vi "AnalyzeLowUpdateData.vi"(8 "error in (no error)":errorcluster, 9 "data in":T12, 11 "Analysis Configuration In":T1 {"Groups"."Calculation Cache"."speed initial conditions"."zoom FFT settings"."FFT settings"."window" items=["Rectangle"=0, "Hanning"=1, "Hamming"=2, "Blackman-Harris"=3, "Exact Blackman"=4, "Blackman"=5, "Flat Top"=6, "4 Term B-Harris "=7, "7 Term B-Harris"=8, "Low Sidelobe"=9, "Blackman Nuttall"=11, "Triangle"=30, "Bartlett-Hanning"=31, "Bohman"=32, "Parzen"=33, "Welch"=34, "Kaiser"=60, "Dolph-Chebyshev"=61, "Gaussian"=62]; "Groups"."Calculation Cache"."spectrum initial conditions"."zoom FFT settings"."FFT settings"."window" items=["Rectangle"=0, "Hanning"=1, "Hamming"=2, "Blackman-Harris"=3, "Exact Blackman"=4, "Blackman"=5, "Flat Top"=6, "4 Term B-Harris "=7, "7 Term B-Harris"=8, "Low Sidelobe"=9, "Blackman Nuttall"=11, "Triangle"=30, "Bartlett-Hanning"=31, "Bohman"=32, "Parzen"=33, "Welch"=34, "Kaiser"=60, "Dolph-Chebyshev"=61, "Gaussian"=62]}) -> (0 "error out":errorcluster, 1 "data out":T12, 3 "Analysis Configuration Out":T1 {"Groups"."Calculation Cache"."speed initial conditions"."zoom FFT settings"."FFT settings"."window" items=["Rectangle"=0, "Hanning"=1, "Hamming"=2, "Blackman-Harris"=3, "Exact Blackman"=4, "Blackman"=5, "Flat Top"=6, "4 Term B-Harris "=7, "7 Term B-Harris"=8, "Low Sidelobe"=9, "Blackman Nuttall"=11, "Triangle"=30, "Bartlett-Hanning"=31, "Bohman"=32, "Parzen"=33, "Welch"=34, "Kaiser"=60, "Dolph-Chebyshev"=61, "Gaussian"=62]; "Groups"."Calculation Cache"."spectrum initial conditions"."zoom FFT settings"."FFT settings"."window" items=["Rectangle"=0, "Hanning"=1, "Hamming"=2, "Blackman-Harris"=3, "Exact Blackman"=4, "Blackman"=5, "Flat Top"=6, "4 Term B-Harris "=7, "7 Term B-Harris"=8, "Low Sidelobe"=9, "Blackman Nuttall"=11, "Triangle"=30, "Bartlett-Hanning"=31, "Bohman"=32, "Parzen"=33, "Welch"=34, "Kaiser"=60, "Dolph-Chebyshev"=61, "Gaussian"=62]})   [LabVIEW 2017, in "McsaAnalysisLowUpdate.lvlib"]
uses:
  <vilib>/addons/InsightCM/Devices/Shared/Mcsa/McsaAnalysisLowUpdate/McsaAnalysisLowUpdate.lvlib
  <vilib>/addons/InsightCM/Devices/Shared/Common/DataFlow/controls/Data.ctl
  <vilib>/addons/InsightCM/Utilities/DataAccessors/controls/wfmSGL_DVR.ctl
  <vilib>/addons/PointValueMap/controls/PointMap.ctl
  <vilib>/addons/InsightCM/Devices/Shared/Common/DataFlow/controls/Type.ctl
  <vilib>/addons/InsightCM/Devices/Shared/Mcsa/McsaAnalysisLowUpdate/controls/Config.ctl
  <vilib>/addons/InsightCM/Devices/Shared/Mcsa/McsaAnalysisLowUpdate/controls/Group.ctl
  <vilib>/addons/InsightCM/Utilities/Analysis/MCSA/controls/McsaLowUpdateChannel.ctl
  <vilib>/addons/InsightCM/Utilities/Analysis/Shared/controls/Feature.ctl
  <vilib>/addons/InsightCM/Utilities/Analysis/Shared/controls/AmplitudeScale.ctl
  <vilib>/addons/InsightCM/Utilities/Analysis/MCSA/controls/McsaMotor.ctl
  <vilib>/addons/InsightCM/Utilities/Analysis/MCSA/controls/McsaCalculationCache.ctl
  <vilib>/addons/Electrical Power/Motor Monitoring/subVIs/ep_Initial Conditions for MCSA Spectra.ctl
  <vilib>/addons/Electrical Power/Motor Monitoring/subVIs/ep_Demodulation Algorithm.ctl
  <vilib>/addons/Electrical Power/Motor Monitoring/subVIs/ep_Zoom FFT Settings.ctl
  <vilib>/addons/Electrical Power/Motor Monitoring/subVIs/ep_Initial Conditions for Speed Estimation.ctl
  <vilib>/addons/InsightCM/Devices/Shared/Mcsa/McsaResourceScheduler/McsaResourceScheduler.lvlib
  <vilib>/addons/PointValueMap/PointValueMap.lvlib
  <vilib>/addons/InsightCM/Devices/Shared/Common/DataFlow/DataFlow.lvlib
  <vilib>/addons/InsightCM/Utilities/Analysis/Shared/AnalysisHelper.lvlib
  <vilib>/addons/InsightCM/Utilities/Analysis/MCSA/McsaAnalysisFunctions.lvlib
  <vilib>/addons/Electrical Power/Motor Monitoring/NI_EP_Motor Monitoring.lvlib
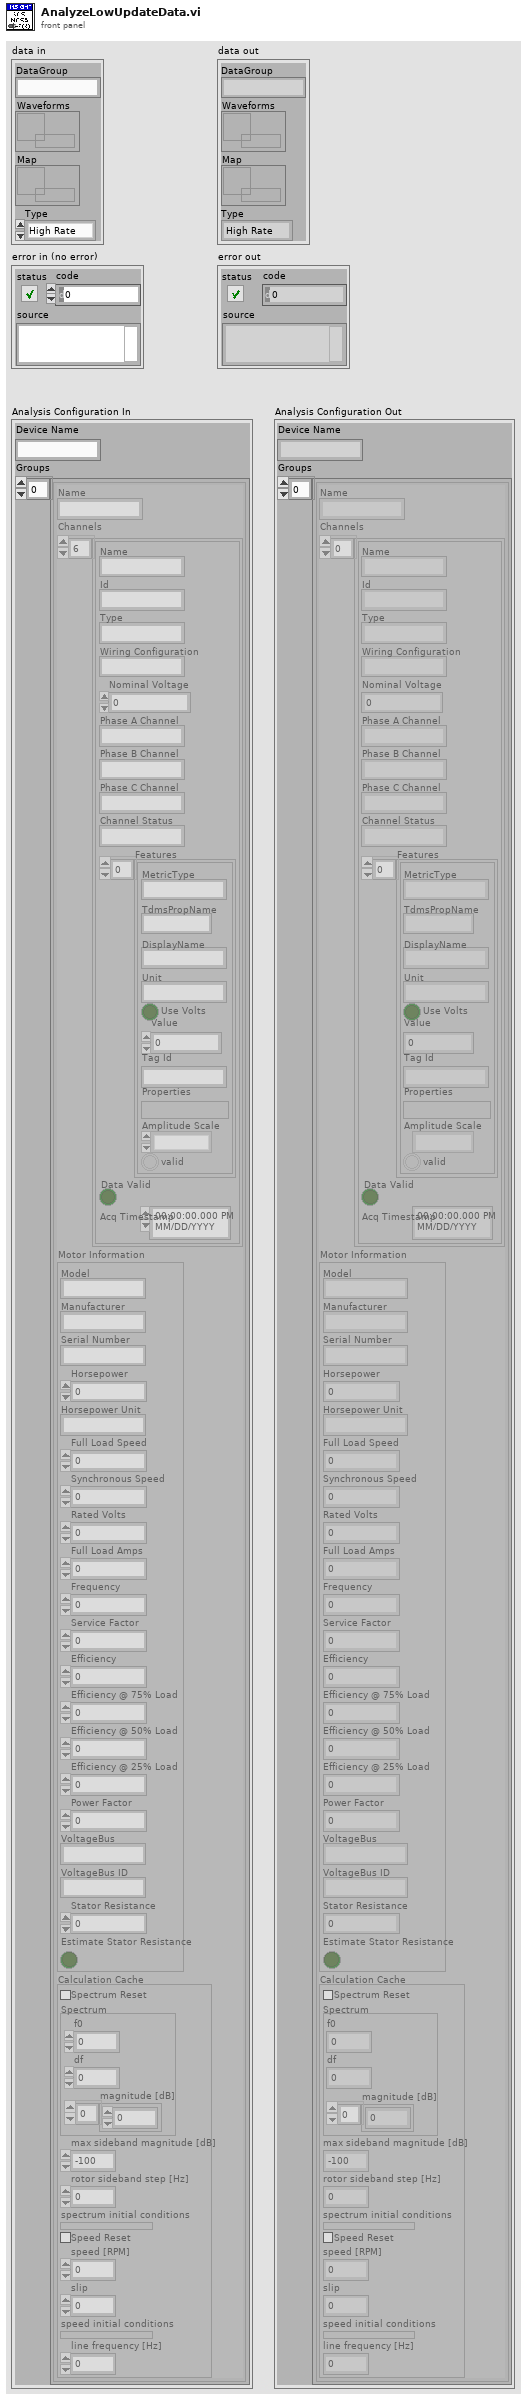
[diagram p1: front panel]
types:
  T1 = typedef "McsaAnalysisLowUpdate.lvlib/Config.ctl" = cluster{"Device Name":string, "Groups":T2[]}
  T2 = typedef "McsaAnalysisLowUpdate.lvlib/Group.ctl" = cluster{"Name":string, "Channels":T3[], "Motor Information":T6, "Calculation Cache":T7}
  T3 = typedef "McsaAnalysisFunctions.lvlib/McsaLowUpdateChannel.ctl" = cluster{"Name":string, "Id":string, "Type":string, "Wiring Configuration":string, "Nominal Voltage":dbl, "Phase A Channel":string, "Phase B Channel":string, "Phase C Channel":string, "Channel Status":string, "Features":T4[], "Data Valid":bool, "Acq Timestamp":timestamp}
  T4 = typedef "AnalysisHelper.lvlib/Feature.ctl" = cluster{"MetricType":string, "TdmsPropName":string, "DisplayName":string, "Unit":string, "Use Volts":bool, "Value":dbl, "Tag Id":string, "Properties":variant, "Amplitude Scale":T5, "valid":bool}
  T5 = typedef "AnalysisHelper.lvlib/AmplitudeScale.ctl" = enum16{"rms", "peak", "pk-pk"}
  T6 = typedef "McsaAnalysisFunctions.lvlib/McsaMotor.ctl" = cluster{"Model":string, "Manufacturer":string, "Serial Number":string, "Horsepower":dbl, "Horsepower Unit":string, "Full Load Speed":dbl, "Synchronous Speed":dbl, "Rated Volts":dbl, "Full Load Amps":dbl, "Frequency":dbl, "Service Factor":dbl, "Efficiency":dbl, "Efficiency @ 75% Load":dbl, "Efficiency @ 50% Load":dbl, "Efficiency @ 25% Load":dbl, "Power Factor":dbl, "VoltageBus":string, "VoltageBus ID":string, "Stator Resistance":dbl, "Estimate Stator Resistance":bool}
  T7 = typedef "McsaAnalysisFunctions.lvlib/McsaCalculationCache.ctl" = cluster{"Spectrum Reset":bool, "Spectrum":cluster{"f0":dbl, "df":dbl, "magnitude [dB]":dbl[]}, "max sideband magnitude [dB]":dbl, "rotor sideband step [Hz]":dbl, "spectrum initial conditions":T8, "Speed Reset":bool, "speed [RPM]":dbl, "slip":dbl, "speed initial conditions":T11, "line frequency [Hz]":dbl}
  T8 = typedef "NI_EP_Motor Monitoring.lvlib/ep_Initial Conditions for MCSA Spectra.ctl" = cluster{"hilbert state":cluster{"delay conditions":dbl[], "filter conditions":dbl[]}, "zoom FFT state":cluster{"phase state":dbl, "zoom FFT state":cluster{"zoom settings state":cluster{"zoom":i32, "stop band attenuation":enum16{"84 dB", "96 dB", "120 dB"}, "alias protect in final transition":bool, "oversampling ratio":dbl}, "SML Decimation Filter (complex input) state":cluster{"decimation settings state":cluster{"M":i32, "stop band attenuation":enum16{"84 dB", "96 dB", "120 dB"}, "alias protect in transition band":bool, "oversampling ratio":dbl}, "counter for garbage samples state":i32, "sml_Parameter Setting for Zoom Factor state":cluster{"filter length * interpolation state":i32, "interpolation state":i32, "comb filter order state":i32, "CFIR par state":cluster{"h":dbl[], "M":i32, "N":i32}, "LFIR par state":cluster{"h":dbl[], "M":i32, "N":i32}, "CIC Stages state":i32}, "aal_CIC (complex input) state":cluster{"aal_cascaded moving average (complex input) state":cluster{"states":cdb[], "circular buffers state":cdb[][], "circular buffer counter state":i32}, "aal_moving average with decimation by order (complex input) state":cluster{"residue result state":cdb, "processed data counter state":i32}}, "sml_Cascaded Decimation Filter (complex input) CFIR state":cluster{"unprocessed data state":cdb[], "final conditions state":cdb[][], "sml_M-1 Decimator with IC (complex input) state":cluster{"coefficients in reverse order state":dbl[], "max index for coefficients state":i32}}, "sml_Cascaded Decimation Filter (complex input) LFIR state":cluster{"unprocessed data state":cdb[], "final conditions state":cdb[][], "sml_M-1 Decimator with IC (complex input) state":cluster{"coefficients in reverse order state":dbl[], "max index for coefficients state":i32}}}, "ma_SML Data Packing (complex input) state":cluster{"array getting packed state":cdb[], "last array processed state":cdb[], "index state":i32, "packing parameters state":cluster{i32, "size":i32}}}, "FFT{X} [Vrms]":cdb[]}, "IIR filter state":cluster{"filter state":dbl[]}, "demodulation settings":cluster{"enable? (F)":bool, "algorithm":T9}, "highpass IIR Filter":cluster{"filter structure":enum32{"IIR 2nd Order", "IIR 4th Order"}, "Reverse Coefficients":dbl[], "Forward Coefficients":dbl[]}, "Hilbert FIR filter":cluster{"coefficients":dbl[], "delay":i32}, "zoom FFT settings":T10}
  T9 = typedef "NI_EP_Motor Monitoring.lvlib/ep_Demodulation Algorithm.ctl" = enum16{"1-phase signal", "3-phase signals"}
  T10 = typedef "NI_EP_Motor Monitoring.lvlib/ep_Zoom FFT Settings.ctl" = cluster{"FFT settings":cluster{"window":u16, "Window Size":i32, "FFT Size":i32, "%overlap":dbl}, "zoom settings":cluster{"zoom":i32, "stop band attenuation":enum16{"84 dB", "96 dB", "120 dB"}, "alias protect in final transition":bool, "oversampling ratio":dbl}, "other settings":cluster{"fmod":dbl, "f0":dbl, "df":dbl, "oidx":i32, "olen":i32}, "iterations":i32, "max block size":i32, "fs":dbl}
  T11 = typedef "NI_EP_Motor Monitoring.lvlib/ep_Initial Conditions for Speed Estimation.ctl" = cluster{"SVAF state":cluster{"space vector amplitude":dbl, "hilbert state":cluster{"delay conditions":dbl[], "filter conditions":dbl[]}}, "zoom FFT state":cluster{"phase state":dbl, "zoom FFT state":cluster{"zoom settings state":cluster{"zoom":i32, "stop band attenuation":enum16{"84 dB", "96 dB", "120 dB"}, "alias protect in final transition":bool, "oversampling ratio":dbl}, "SML Decimation Filter (complex input) state":cluster{"decimation settings state":cluster{"M":i32, "stop band attenuation":enum16{"84 dB", "96 dB", "120 dB"}, "alias protect in transition band":bool, "oversampling ratio":dbl}, "counter for garbage samples state":i32, "sml_Parameter Setting for Zoom Factor state":cluster{"filter length * interpolation state":i32, "interpolation state":i32, "comb filter order state":i32, "CFIR par state":cluster{"h":dbl[], "M":i32, "N":i32}, "LFIR par state":cluster{"h":dbl[], "M":i32, "N":i32}, "CIC Stages state":i32}, "aal_CIC (complex input) state":cluster{"aal_cascaded moving average (complex input) state":cluster{"states":cdb[], "circular buffers state":cdb[][], "circular buffer counter state":i32}, "aal_moving average with decimation by order (complex input) state":cluster{"residue result state":cdb, "processed data counter state":i32}}, "sml_Cascaded Decimation Filter (complex input) CFIR state":cluster{"unprocessed data state":cdb[], "final conditions state":cdb[][], "sml_M-1 Decimator with IC (complex input) state":cluster{"coefficients in reverse order state":dbl[], "max index for coefficients state":i32}}, "sml_Cascaded Decimation Filter (complex input) LFIR state":cluster{"unprocessed data state":cdb[], "final conditions state":cdb[][], "sml_M-1 Decimator with IC (complex input) state":cluster{"coefficients in reverse order state":dbl[], "max index for coefficients state":i32}}}, "ma_SML Data Packing (complex input) state":cluster{"array getting packed state":cdb[], "last array processed state":cdb[], "index state":i32, "packing parameters state":cluster{i32, "size":i32}}}, "FFT{X} [Vrms]":cdb[]}, "speed state":cluster{"speed [RPM]":dbl, "slip":dbl}, "speed estimation settings":cluster{"% overlap":dbl, "algorithm":T9}, "filter information":cluster{"coefficients":dbl[], "order":i32}, "zoom FFT settings":T10, "last valid window":i32, "fund. frequency for averager":dbl[]}
  T12 = typedef "DataFlow.lvlib/Data.ctl" = cluster{"DataGroup":string, "Waveforms":T13, "Map":T14, "Type":T15}
  T13 = typedef "wfmSGL_DVR.ctl" = refnum<data-value>
  T14 = typedef "PointValueMap.lvlib/PointMap.ctl" = refnum<data-value>
  T15 = typedef "DataFlow.lvlib/Type.ctl" = enum16{"High Rate", "Low Rate", "Burst Mode"}
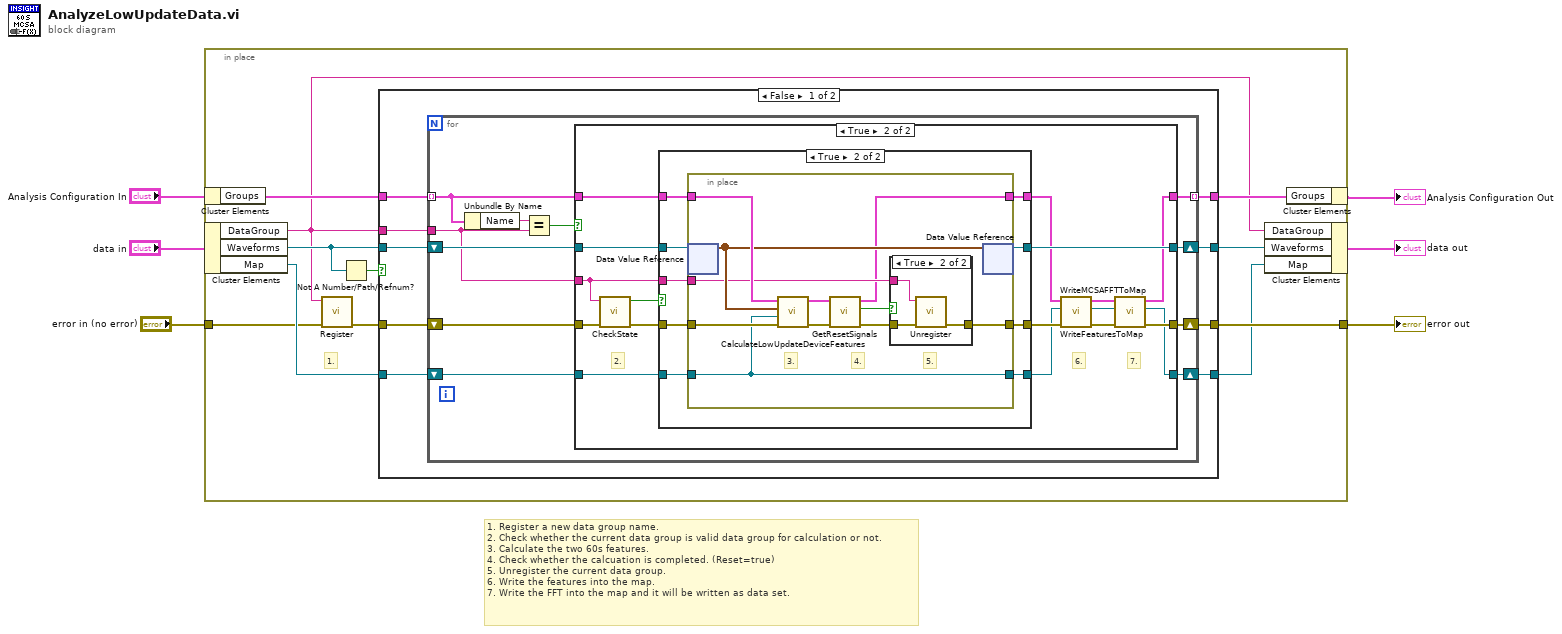
[diagram p0: block diagram]
diagram:
  # "1. Register a new data group name.\n2. Check whether the current data group is valid data group for calculation or not.\n3. Calculate the two 60s features.\n4. Check whether the calcuation is completed. (Reset=true)\n5. Unregister the current data group.\n6. Write the features into the map.\n7. Write the FFT into the map and it will be written as data set."
  n1 = in-place {
    in-place-border: [w17] -> w3
    in-place-border: "error in (no error)" -> [w9]
    # "1."
    n2 = in-place-cluster #1("Analysis Configuration In") -> ("Groups"=w16:T2[])
    n3 = in-place-cluster #2("data in") -> ("DataGroup"=w7:string, "Waveforms"=w11:T13, "Map"=w14:T14)
    n4 = call <vilib>:"Register.vi"("error in (no error)"=w9, "name"=w7) -> ("error out"=w8:errorcluster)  [unwired: 9 in]
    n5 = Not A Number/Path/Refnum?(number/path/refnum=w11) -> (NaN/Path/Refnum?=w10:bool)
    n6 = case shown="False" w10 {
      tunnel: [w26 w87] -> w17
      tunnel: w16 -> [w25 w89]
      tunnel: [w24 w89] -> w15
      tunnel: w8 -> [w23 w87]
      tunnel: w14 -> [w22 w86]
      tunnel: [w21 w88] -> w13
      tunnel: w7 -> [w20 _]
      tunnel: [w19 w86] -> w12
      tunnel: w11 -> [w18 w88]
      frame False {
        n7 = for {
          tunnel: w20 -> [w28]
          shift-right: [w31] -> w26
          shift-left: w23 -> [w32]
          tunnel: w25 -> [w34] mode=indexing
          tunnel: [w30] -> w24 mode=indexing
          shift-right: [w33] -> w21
          shift-left: w18 -> [w37]
          shift-right: [w29] -> w19
          shift-left: w22 -> [w36]
          n8 = Unbundle By Name(w34) -> ("Name"=w35:string)
          n9 = Equal?(x=w35, y=w28) -> (x = y?=w27:bool)
          n10 = case shown="True" w27 {
            tunnel: w37 -> [w40 w58]
            tunnel: w36 -> [w38 w57]
            tunnel: w34 -> [w41 w56]
            tunnel: [w40 w55] -> w33
            tunnel: w32 -> [w39 w54]
            tunnel: [w39 w48] -> w31
            tunnel: [w41 w45] -> w30
            tunnel: [w38 w44] -> w29
            tunnel: w28 -> [_ w42]
            frame False {
            }
            frame True {
              # "7."
              # "6."
              # "2."
              n11 = call <vilib>:"CheckState.vi"("error in (no error)"=w54, "name"=w42) -> ("error out"=w53:errorcluster, "active"=w43:bool)  [unwired: 8 in]
              n12 = case shown="True" w43 {
                tunnel: [w61 w71] -> w52
                tunnel: w58 -> [w60 w70]
                tunnel: w57 -> [w59 w69]
                tunnel: w53 -> [w61 w68]
                tunnel: w56 -> [w62 w67]
                tunnel: [w62 w66] -> w50
                tunnel: [w60 w65] -> w55
                tunnel: [w59 w64] -> w51
                tunnel: w42 -> [_ w63]
                frame False {
                }
                frame True {
                  n13 = in-place {
                    in-place-border: w68 -> [w79]
                    in-place-border: [w78] -> w71
                    in-place-border: [w72] -> w66
                    in-place-border: w69 -> [w75]
                    in-place-border: w67 -> [w81]
                    in-place-border: [w75] -> w64
                    in-place-border: w63 -> [w73]
                    # "5."
                    # "4."
                    # "3."
                    n14 = in-place-dvr #3(w70) -> (w80:waveform(sgl)[])  [unwired: 1 out]
                    n15 = call <vilib>:"CalculateLowUpdateDeviceFeatures.vi"("error in (no error)"=w79, "data flow map in"=w75, "Waveforms"=w80, "Group in"=w81) -> ("error out"=w76:errorcluster, "Group out"=w74:T2)  [unwired: 6 in]
                    n16 = call <vilib>:"GetResetSignals.vi"("Group in"=w74) -> ("Reset?"=w77:bool, "Group out"=w72:T2)  [unwired: 9 in]
                    n17 = case shown="True" w77 {
                      tunnel: w76 -> [w82 w85]
                      tunnel: [w82 w84] -> w78
                      tunnel: w73 -> [_ w83]
                      frame False {
                      }
                      frame True {
                        n18 = call <vilib>:"Unregister.vi"("error in (no error)"=w85, "name"=w83) -> ("error out"=w84:errorcluster)  [unwired: 9 in]
                      }
                    }
                    n19 = in-place-dvr #3(w80) -> (w65:T13)  [unwired: 1 out]
                  }
                }
              }
              n20 = call <vilib>:"WriteFeaturesToMap.vi"("error in (no error)"=w52, "Map in"=w51, "Group"=w50) -> ("error out"=w49:errorcluster, "Map out"=w47:T14, "Group out"=w46:T2)  [unwired: 6 in]
              n21 = call <vilib>:"WriteMCSAFFTToMap.vi"("error in (no error)"=w49, "Map in"=w47, "Group in"=w46) -> ("error out"=w48:errorcluster, "Map out"=w44:T14, "Group out"=w45:T2)  [unwired: 6 in]
            }
          }
        }
      }
      frame True {
      }
    }
    n22 = in-place-cluster #2("DataGroup"=w7, "Waveforms"=w13, "Map"=w12) -> (→"data out":T12)
    n23 = in-place-cluster #1("Groups"=w15) -> (→"Analysis Configuration Out":T1)
  }
  "error out" <- w3
